vi "AWG.vi"(9 "ampiezza":dbl, 10 "frequenza":dbl, 11 "tipo":enum16{"sin", "squ", "tri"}(ring)) -> ()   [LabVIEW 2013]
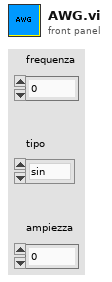
[diagram p1: front panel]
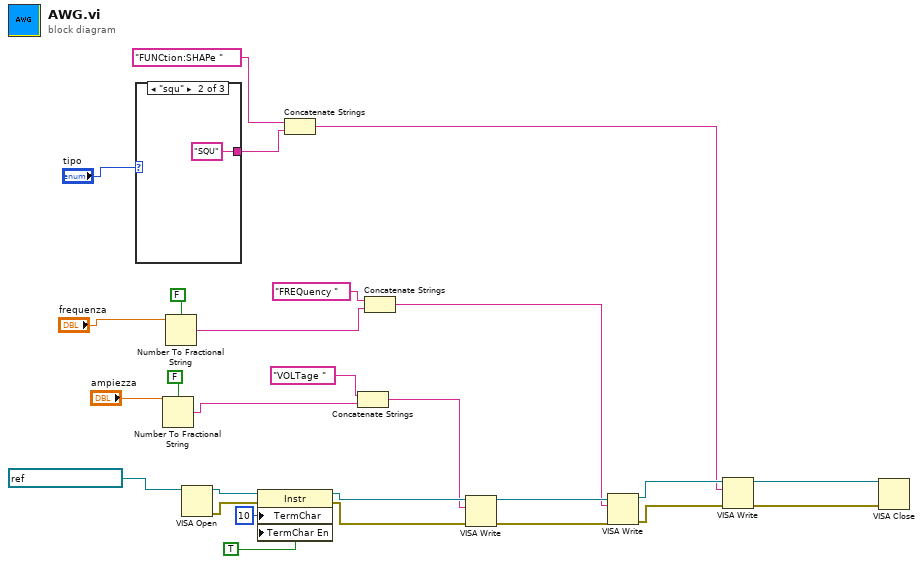
[diagram p0: block diagram]
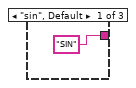
[diagram p2: hidden frame]
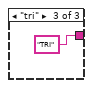
[diagram p3: hidden frame]
diagram:
  n1 = case shown="\"squ\"" "tipo" {
    tunnel: ["SIN" "SQU" "TRI"] -> w25
    frame "sin", Default {
    }
    frame "squ" {
    }
    frame "tri" {
    }
  }
  n2 = Number To Fractional String(use system decimal point (T)=FALSE, number="ampiezza") -> (F-format string=w17:string)  [unwired: 2 in]
  n3 = Number To Fractional String(use system decimal point (T)=FALSE, number="frequenza") -> (F-format string=w19:string)  [unwired: 2 in]
  n4 = VISA Open(VISA resource name=refnum<visa-resource-name> "GPIB0::23::INSTR") -> (VISA resource name=w15:refnum<visa-resource-name>, error out=w14:errorcluster)  [unwired: 4 in]
  n5 = property class="Instr"(reference=w15, error in=w14, "TermChar"=u8 10 ("Message Based Settings:Termination Character"), "TermChar En"=TRUE ("Message Based Settings:Termination Character Enable")) -> (reference out=w9:refnum<visa-resource-name>, error out=w4:errorcluster)
  n6 = Concatenate Strings("FUNCtion:SHAPe ", w25) -> (w3:string)
  n7 = Concatenate Strings("VOLTage ", w17) -> (w1:string)
  n8 = Concatenate Strings("FREQuency ", w19) -> (w2:string)
  n9 = VISA Write(VISA resource name=w9, write buffer=w1, error in (no error)=w4) -> (VISA resource name out=w8:refnum<visa-resource-name>, error out=w5:errorcluster)  [unwired: 1 out]
  n10 = VISA Write(VISA resource name=w8, write buffer=w2, error in (no error)=w5) -> (VISA resource name out=w7:refnum<visa-resource-name>, error out=w6:errorcluster)  [unwired: 1 out]
  n11 = VISA Write(VISA resource name=w7, write buffer=w3, error in (no error)=w6) -> (VISA resource name out=w11:refnum<visa-resource-name>, error out=w10:errorcluster)  [unwired: 1 out]
  n12 = VISA Close(VISA resource name=w11, error in (no error)=w10) -> ()  [unwired: 1 out]
